vi "GetPositiveFixInt.vi"(8 "error in (no error)":errorcluster, 11 "MsgPackDeserializer in":refnum<class "MsgPackDeserializer.lvclass">) -> (0 "error out":errorcluster, 2 "Number":u8, 3 "MsgPackDeserializer out":refnum<class "MsgPackDeserializer.lvclass">)   [LabVIEW 2015, in "MsgPackDeserializer.lvclass"]
uses:
  MsgPackDeserializer.lvclass
  MsgPackDeserializer.lvclass/MsgPackDeserializer.ctl
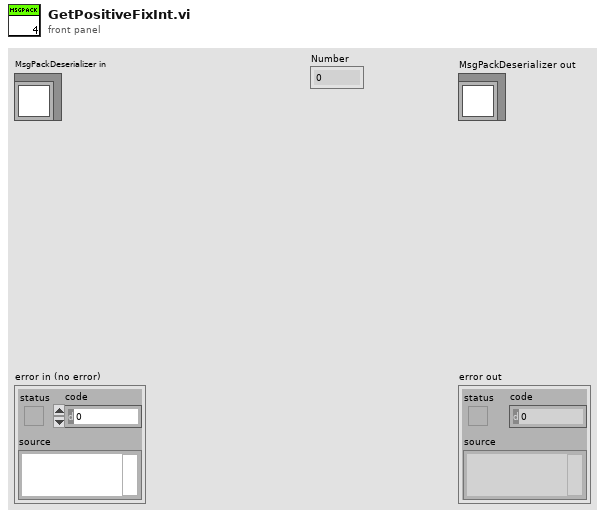
[diagram p1: front panel]
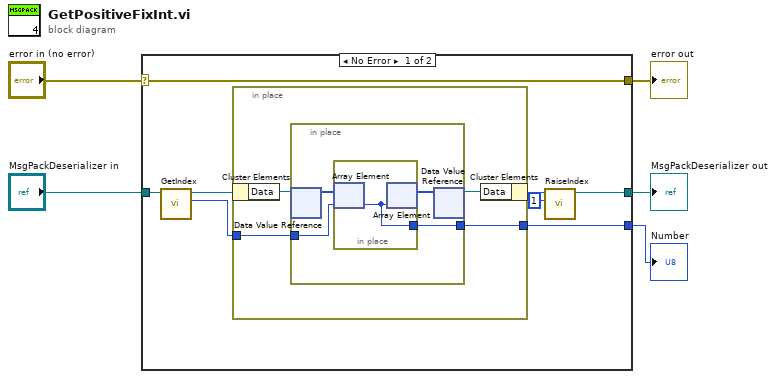
[diagram p0: block diagram]
diagram:
  n1 = case shown="No Error" "error in (no error)" {
    selector: "error in (no error)" -> [w13 w24]
    tunnel: [w13 w24] -> w4
    tunnel: [w9 w23] -> w2
    tunnel: "MsgPackDeserializer in" -> [w12 w23]
    tunnel: [w7 _] -> w1
    frame No Error {
      n2 = call "GetIndex.vi"("MsgPackDeserializer in"=w12) -> ("Index"=w10:i64, "MsgPackDeserializer out"=w11:refnum<class "MsgPackDeserializer.lvclass">)  [unwired: 8 in, 1 out]
      n3 = in-place {
        in-place-border: [w16] -> w7
        in-place-border: w10 -> [w15]
        n4 = in-place-cluster #1(w11) -> ("Data"=w14:refnum<data-value>)
        n5 = in-place {
          in-place-border: [w21] -> w16
          in-place-border: w15 -> [w20]
          n6 = in-place-dvr #2(w14) -> (w19:u8[])  [unwired: 1 out]
          n7 = in-place {
            in-place-border: [w22] -> w21
            n8 = in-place-array #3(w19, w20) -> (w22:u8)
            n9 = in-place-array #3(w22) -> (w18:u8[])  [unwired: 1 out]
          }
          n10 = in-place-dvr #2(w18) -> (w17:refnum<data-value>)  [unwired: 1 out]
        }
        n11 = in-place-cluster #1("Data"=w17) -> (w8:refnum<class "MsgPackDeserializer.lvclass">)
      }
      n12 = call "RaiseIndex.vi"("x"=i64 1, "MsgPackDeserializer in"=w8) -> ("MsgPackDeserializer out"=w9:refnum<class "MsgPackDeserializer.lvclass">)  [unwired: 8 in, 1 out]
    }
    frame Error {
    }
  }
  "error out" <- w4
  "MsgPackDeserializer out" <- w2
  "Number" <- w1
